vi "Apply Configuration.vi"(8 "error in":errorcluster, 11 "IConfigurable in":refnum<class "IConfigurable.lvclass">) -> (0 "error out":errorcluster, 3 "IConfigurable out":refnum<class "IConfigurable.lvclass">)   [LabVIEW 2025, in "IConfigurable.lvclass"]
uses:
  IConfigurable.lvclass
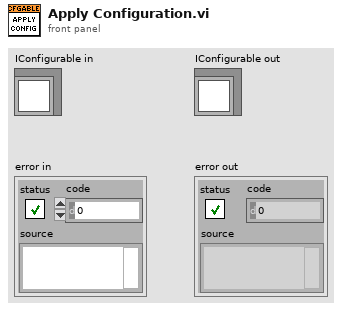
[diagram p1: front panel]
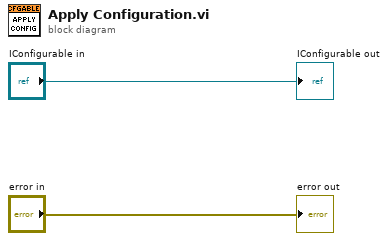
[diagram p0: block diagram]
diagram:
  "error out" <- "error in"
  "IConfigurable out" <- "IConfigurable in"
